vi "Easy Write XML File.vi"(5 "Encoding (none)":string, 6 "Standalone? (true)":bool=TRUE, 7 "Stylesheet URL (none)":string, 8 "error in (no error)":errorcluster, 9 "Overwrite File? (false)":bool, 10 "LabVIEW Data":variant, 11 "XML File Path":path) -> (0 "error out":errorcluster, 3 "XML File Path (duplicate)":path)   [LabVIEW 2013]
doc: "Converts <B>LabVIEW Data</B> to an XML string and writes it to an XML file with the LabVIEW data names (labels) converted to XML item names and the LabVIEW data values converted to XML item values."
uses:
  <userlib>/_OpenG.lib/lvdata/lvdata.llb/Type Descriptor Enumeration__ogtk.ctl
  <userlib>/_OpenG.lib/file/file.llb/File Exists - Scalar__ogtk.vi
panel:
  # "JKI EasyXML Toolkit for LabVIEW\nhttp://jki.net/easyxml\nCopyright (C) 2007-2016, JKI <info@jki.net>\nALL RIGHTS RESERVED"
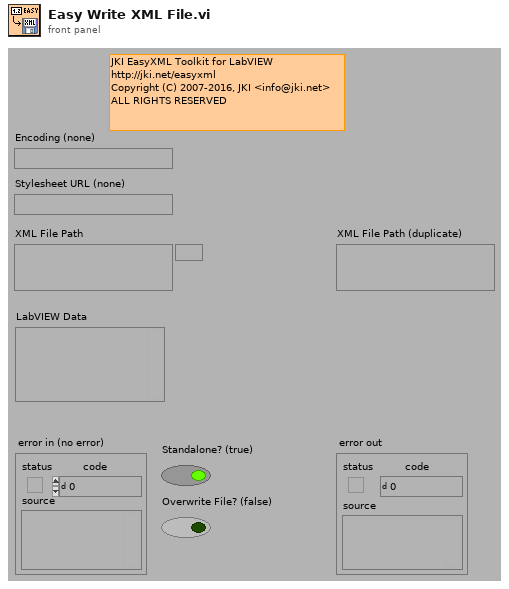
[diagram p1: front panel]
types:
  T1 = enum16{"open", "replace", "create", "open or create", "replace or create", "replace or create with confirmation"}
  T2 = typedef "Type Descriptor Enumeration__ogtk.ctl" = enum8{"<Null>", "I8", "I16", "I32", "I64", "U8", "U16", "U32", "U64", "SGL", "DBL", "EXT", "CSG", "CDB", "CXT", "0x0F", "0x10", "0x11", "0x12", "0x13", "0x14", "Enum U8", "Enum U16", "Enum U32", "Enum U64", "SGL PQ", "DBL PQ", "EXT PQ", "CSG PQ", "CDB PQ", "CXT PQ", "0x1F", "0x20", "Boolean", "0x22", "0x23", "0x24", "0x25", "0x26", "0x27", "0x28", "0x29", "0x2A", "0x2B", "0x2C", "0x2D", "0x2E", "0x2F", "String", "0x31", "Path", "Pict", "0x34", "0x35", "0x36", "DAQ", "0x38", "0x39", "0x3A", "0x3B", "0x3C", "0x3D", "0x3E", "0x3F", "Array", "0x41", "0x42", "0x43", "0x44", "0x45", "0x46", "0x47", "0x48", "0x49", "0x4A", "0x4B", "0x4C", "0x4D", "0x4E", "0x4F", "Cluster", "0x51", "0x52", "Variant", "Waveform", "0x55", "0x56", "0x57", "0x58", "0x59", "0x5A", "0x5B", "0x5C", "0x5D", "0x5E", "0x5F", "0x60", "0x61", "0x62", "0x63", "0x64", "0x65", "0x66", "0x67", "0x68", "0x69", "0x6A", "0x6B", "0x6C", "0x6D", "0x6E", "0x6F", "Refnum"}
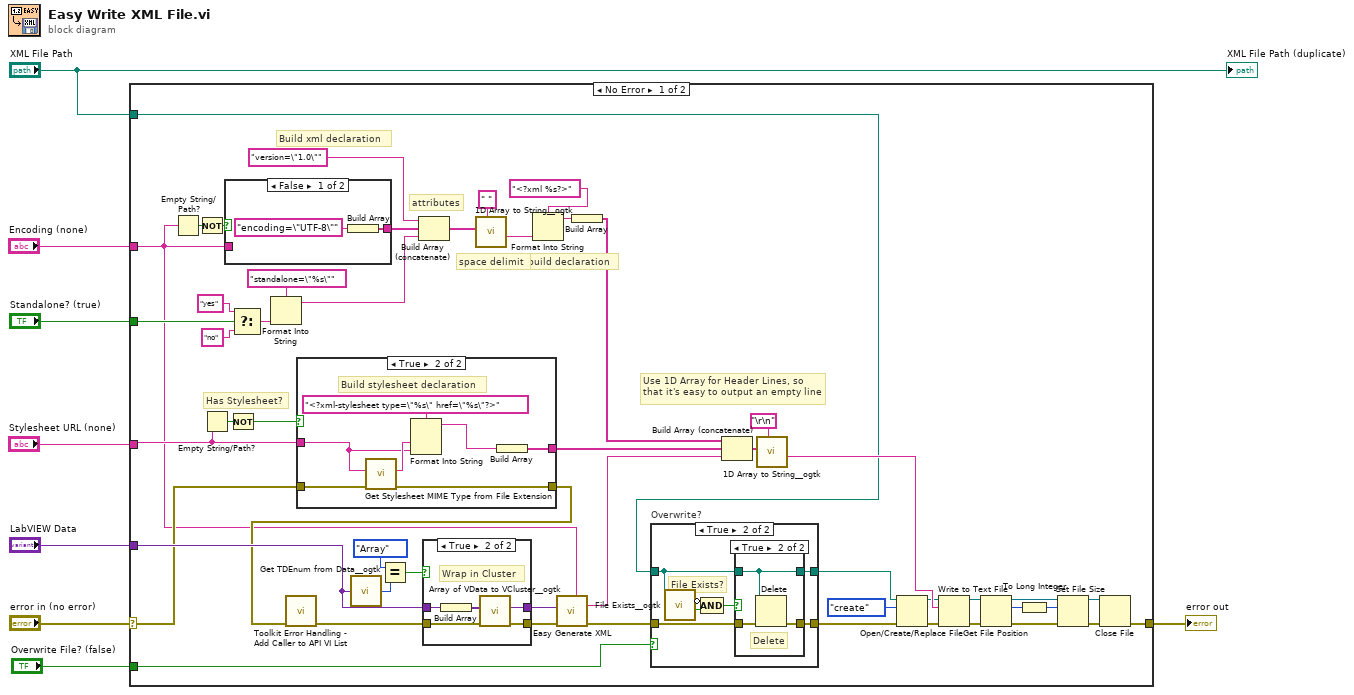
[diagram p0: block diagram]
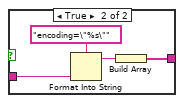
[diagram p4: hidden frame]
diagram:
  n1 = case shown="No Error" "error in (no error)" {
    selector: "error in (no error)" -> [w40 w95]
    tunnel: [w47 w95] -> w7
    tunnel: "LabVIEW Data" -> [w54 _]
    tunnel: "XML File Path" -> [w11 _]
    tunnel: "Stylesheet URL (none)" -> [w52 _]
    tunnel: "Encoding (none)" -> [w9 _]
    tunnel: "Standalone? (true)" -> [w50 _]
    tunnel: "Overwrite File? (false)" -> [w12 _]
    frame No Error {
      # "Use 1D Array for Header Lines, so that it's easy to output an empty line"
      # "build declaration"
      # "space delimit"
      # "attributes"
      # "Build xml declaration"
      # "Has Stylesheet?"
      n2 = Empty String/Path?(string/path=w9) -> (empty?=w24:bool)
      n3 = Not(x=w24) -> (.not. x?=w22:bool)
      n4 = Empty String/Path?(string/path=w52) -> (empty?=w51:bool)
      n5 = case shown="False" w22 {
        tunnel: w9 -> [_ w78]
        tunnel: [w74 w76] -> w23
        frame False {
          n6 = Build Array("encoding=\"UTF-8\"") -> (w74:string[])
        }
        frame True {
          n7 = Format Into String(format string="encoding=\"%s\"", w78) -> (resulting string=w77:string)  [unwired: 2 in, 1 out]
          n8 = Build Array(w77) -> (w76:string[])
        }
      }
      n9 = Not(x=w51) -> (.not. x?=w41:bool)
      n10 = Select(t="yes", s=w50, f="no") -> (s? t:f=w27:string)
      n11 = Format Into String(format string="standalone=\"%s\"", w27) -> (resulting string=w25:string)  [unwired: 2 in, 1 out]
      n12 = case shown="True" w41 {
        tunnel: w52 -> [_ w81]
        tunnel: [_ w84] -> w32
        tunnel: [w80 w86] -> w39
        tunnel: w40 -> [w80 w85]
        frame False {
        }
        frame True {
          # "Build stylesheet declaration"
          n13 = call "Get Stylesheet MIME Type from File Extension.vi"("error in"=w85, "Stylesheet URL"=w81) -> ("error out"=w86:errorcluster, "MIME type"=w82:string)  [unwired: 8 in]
          n14 = Format Into String(format string="<?xml-stylesheet type=\"%s\" href=\"%s\"?>", w82, w81) -> (resulting string=w83:string)  [unwired: 2 in, 1 out]
          n15 = Build Array(w83) -> (w84:string[])
        }
      }
      n16 = call "Toolkit Error Handling - Add Caller to API VI List.vi"("error in"=w39) -> ("error out"=w53:errorcluster)  [unwired: 10 in]
      n17 = call <userlib>:"Get TDEnum from Data__ogtk.vi"("Data"=w54) -> ("Type Descriptor Enumeration"=w59:T2)  [unwired: 4 in]
      n18 = Equal?(x=Type_Descriptor_Enumeration__ogtk."Array" ("Type Descriptor Enumeration"), y=w59) -> (x = y?=w57:bool)
      n19 = Build Array (concatenate)("version=\"1.0\"", w23, w25) -> (w37:string[])
      n20 = case shown="True" w57 {
        tunnel: w53 -> [w89 w93]
        tunnel: [w89 w92] -> w56
        tunnel: w54 -> [w88 w91]
        tunnel: [w88 w90] -> w55
        frame False {
        }
        frame True {
          # "Wrap in Cluster"
          n21 = Build Array(w91) -> (w94:variant[])
          n22 = call <userlib>:"Array of VData to VCluster__ogtk.vi"("error in (no error)"=w93, "Array"=w94) -> ("error out"=w92:errorcluster, "VCluster"=w90:variant)  [unwired: 8 in]
        }
      }
      n23 = call <userlib>:"1D Array to String__ogtk.vi"("delimiter (Tab)"=" ", "Array of Strings"=w37) -> ("delimited string"=w35:string)  [unwired: 9 in]
      n24 = Format Into String(format string="<?xml %s?>", w35) -> (resulting string=w33:string)  [unwired: 2 in, 1 out]
      n25 = call "Easy Generate XML.vi"("Encoding (none)"=w9, "error in (no error)"=w56, "LabVIEW Data"=w55) -> ("error out"=w14:errorcluster, "XML String"=w30:string)  [unwired: 7 in]
      n26 = Build Array(w33) -> (w19:string[])
      n27 = case "Overwrite?" shown="True" w12 {
        tunnel: [w61 w62] -> w13
        tunnel: w14 -> [w61 w65]
        tunnel: w11 -> [w60 w64]
        tunnel: [w60 w63] -> w10
        frame False {
        }
        frame True {
          # "File Exists?"
          n28 = call-poly <userlib>:"File Exists__ogtk.vi"("file path"=w64) -> ("is directory"=w68:bool, "exists"=w67:bool)  [unwired: 6 in]
          n29 = Compound Arithmetic op=AND(invert w68, w67) -> (w66:bool)
          n30 = case shown="True" w66 {
            tunnel: w65 -> [w69 w73]
            tunnel: w64 -> [w70 w72]
            tunnel: [w70 w72] -> w63
            tunnel: [w69 w71] -> w62
            frame False {
            }
            frame True {
              # "Delete"
              n31 = Delete(path (use dialog)=w72, error in=w73) -> (error out=w71:errorcluster)  [unwired: 3 in, 2 out]
            }
          }
        }
      }
      n32 = Build Array (concatenate)(w19, w32, w30) -> (w31:string[])
      n33 = call <userlib>:"1D Array to String__ogtk.vi"("delimiter (Tab)"="\r\n", "Array of Strings"=w31) -> ("delimited string"=w29:string)  [unwired: 9 in]
      n34 = Open/Create/Replace File(file path (use dialog)=w10, error in=w13, operation (0:open)=T1."create") -> (refnum out=w20:refnum<file>, error out=w21:errorcluster)  [unwired: 3 in, 1 out]
      n35 = Write to Text File(file (use dialog)=w20, text=w29, error in=w21) -> (refnum out=w17:refnum<file>, error out=w16:errorcluster)  [unwired: 1 in, 1 out]
      n36 = Get File Position(4:w16, 7:w17) -> (0:w46:errorcluster, 2:w15:i64, 3:w45:refnum<file>)
      n37 = To Long Integer(number=w15) -> (32bit integer=w42:i32)
      n38 = Set File Size(4:w46, 6:w42, 7:w45) -> (0:w43:errorcluster, 3:w44:refnum<file>)
      n39 = Close File(refnum=w44, error in=w43) -> (error out=w47:errorcluster)  [unwired: 1 out]
    }
    frame Error {
    }
  }
  "error out" <- w7
  "XML File Path (duplicate)" <- "XML File Path"
